vi "Meadowlark USB IO Example_2.VI"(0 "Set Voltage":dbl min=0.0 max=10.0 step=0.001 format="%.3f", 5 "error in (no error)":errorcluster) -> (14 "Readout \nVoltages":dbl[](array[numeric]) format="%.3f", 19 "error out":errorcluster)   [LabVIEW 2017]
doc: "This example selects channels and sets and reads voltages on a Meadowlark Optics D3040 Four-Cell controller. This VI can be opened and examined using LabVIEW (6.1 or newer) as a starting point for a user's custom development of a D3040 interface. Please note that the Sub-VI's used in this program require the file \"usbdrvd.dll\".\n\n(c) 2002-2003 Meadowlark Optics, Inc. All rights reserved."
panel:
  out "FW Version":dbl=2.0 min=0.0 max=10.0 step=0.001 format="%.2f"
  out "Update \nChannel":bool[](array[boolean])
  out "Located USB Devices":bool[](array[boolean])=[TRUE]
  in  "USB Device Number":i32=1 min=0 max=0
  in  "Channel":i32=2 min=1 max=4 step=1
  # "1"
  # "2"
  # "3"
  # "4"
  # "5"
  # "6"
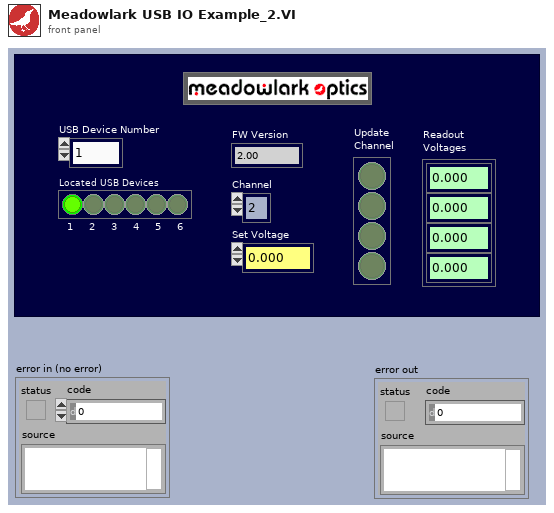
[diagram p1: front panel]
types:
  T1 = cluster{"Device Handle":u32, "Pipe 0 Handle":u32, "Pipe 1 Handle":u32}[]
  T2 = cluster{"Device Handle":u32, "Pipe 0 Handle":u32, "Pipe 1 Handle":u32}
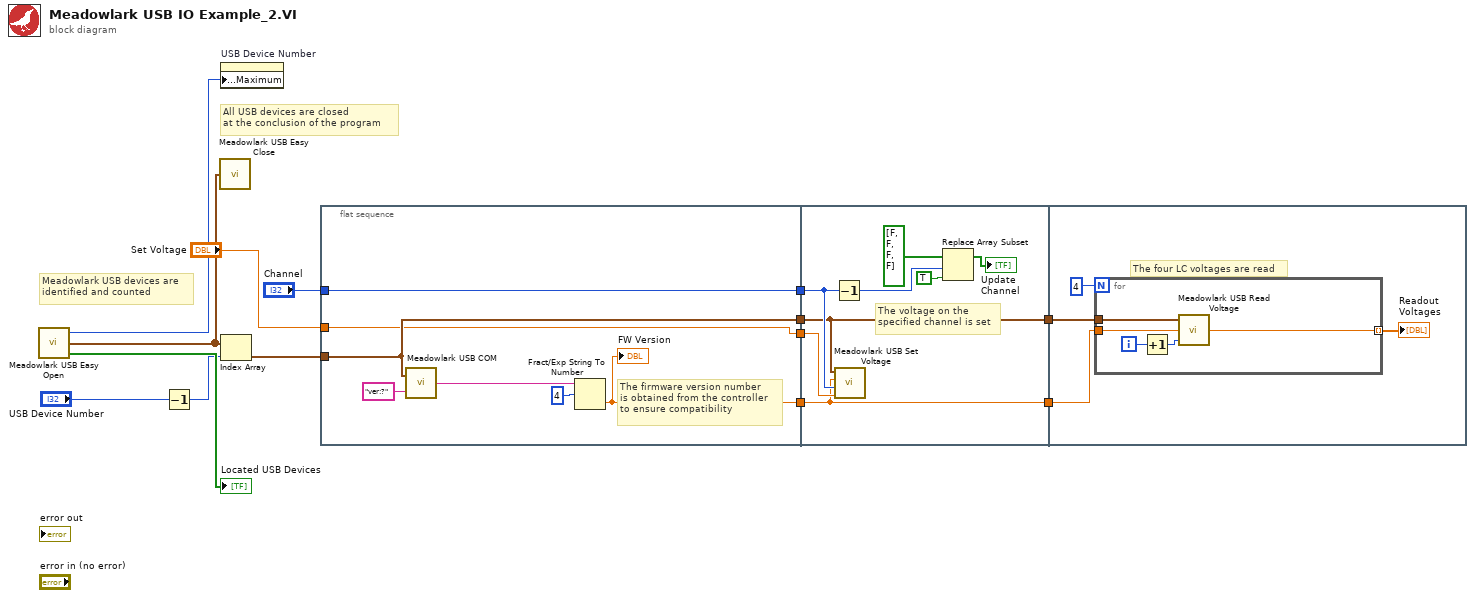
[diagram p0: block diagram]
diagram:
  # "All USB devices are closed\nat the conclusion of the program"
  # "Meadowlark USB devices are\nidentified and counted"
  n1 = call "Meadowlark USB Easy Open.vi"() -> ("Device Opened Array"=→"Located USB Devices":bool[], "USB Device and Pipes Array"=w14:T1, "Device Count"=w13:u32)
  n2 = Decrement(x="USB Device Number") -> (x-1=w9:i32)
  n3 = call "Meadowlark USB Easy Close.vi"("USB Device and Pipes Array"=w14) -> ()
  n4 = property on="USB Device Number" class="DigNum (strict)"("Data Entry Limits:Maximum"=w13) -> ()  [unwired: 2 in, 2 out]
  n5 = Index Array(array=w14, index=w9) -> (element=w7:T2)
  n6 = flat-sequence {
    tunnel: "Set Voltage" -> [w16]
    tunnel: [w16] -> w6
    tunnel: "Channel" -> [w15]
    tunnel: [w15] -> w5
    tunnel: w7 -> [w21]
    tunnel: [w21] -> w4
    tunnel: [w17] -> w3
    tunnel: w6 -> [w29]
    tunnel: w5 -> [w25]
    tunnel: w4 -> [w23]
    tunnel: [w23] -> w2
    tunnel: w3 -> [w22]
    tunnel: [w22] -> w1
    tunnel: w2 -> [w31]
    tunnel: w1 -> [w30]
    frame #0 {
      # "The firmware version number\nis obtained from the controller\nto ensure compatibility"
      n7 = call "Meadowlark USB COM.vi"("WRITE IN String"="ver:?", "USB Open Device Cluster"=w21) -> ("READ OUT String"=w19:string)
      n8 = Fract/Exp String To Number(string=w19, offset=4) -> (number=w17:dbl)  [unwired: 2 in, 1 out]
      "FW Version" <- w17
    }
    frame #1 {
      # "The voltage on the\nspecified channel is set"
      n9 = Decrement(x=w25) -> (x-1=w28:i32)
      n10 = call "Meadowlark USB Set Voltage.VI"("LC Voltage"=w29, "LC Channel"=w25, "FW Version"=w22, "USB Open Device Cluster"=w23) -> ()  [unwired: 1 out]
      n11 = Replace Array Subset(array=bool[] [FALSE, FALSE, FALSE, FALSE], new element=TRUE ("new element/subarray"), index=w28) -> (→"Update \nChannel":bool[])
    }
    frame #2 {
      # "The four LC voltages are read"
      n12 = for {
        N: 4 -> [_]
        tunnel: [w37] -> w32 mode=indexing
        tunnel: w31 -> [w36]
        tunnel: w30 -> [w34]
        i -> [w38]
        n13 = Increment(x=w38) -> (x+1=w35:i32)
        n14 = call "Meadowlark USB Read Voltage.VI"("LC Channel"=w35, "FW Version"=w34, "USB Open Device Cluster"=w36) -> ("Readout \nVoltage"=w37:dbl)
      }
      "Readout \nVoltages" <- w32
    }
  }
